vi "TPS Global.vi"() -> ()   [LabVIEW 2009]
doc: "This Global is written to by TPS System Start."
panel:
  in  "TPS Setup File":string="DEM103_Setup_File.txt"
  in  "TPS Base Path":path=path "D:/Documents and Settings/All Users/Desktop/NMR program/NMR program"
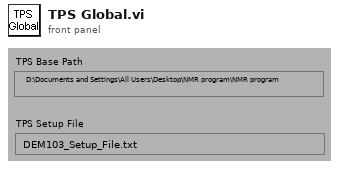
[diagram p1: front panel]
diagram:
